vi "Controller - Fire Emergency.vi"(8 "error in (no error)":errorcluster, 10 "Emergency":bool, 11 "View Model":T1) -> (0 "error out":errorcluster, 3 "View Model":T1)   [LabVIEW 2017]
doc: "Fire User Event = Emergency"
uses:
  View Model/Controls/View Model.ctl
  View Model/Controls/Shared Model.ctl
  Error/Controls/Error Model.ctl
  Error/Controls/Error Event.ctl
  Error/Controls/Error Type.ctl
  Configuration/Controls/Config DB Model.ctl
  Configuration/Controls/Config DB Command.ctl
  Configuration/Controls/Config DB Record.ctl
  Controls/Controller Model.ctl
  Controls/Elevator Location.ctl
  Controls/Elevator Direction Event.ctl
  Controls/Elevator Direction.ctl
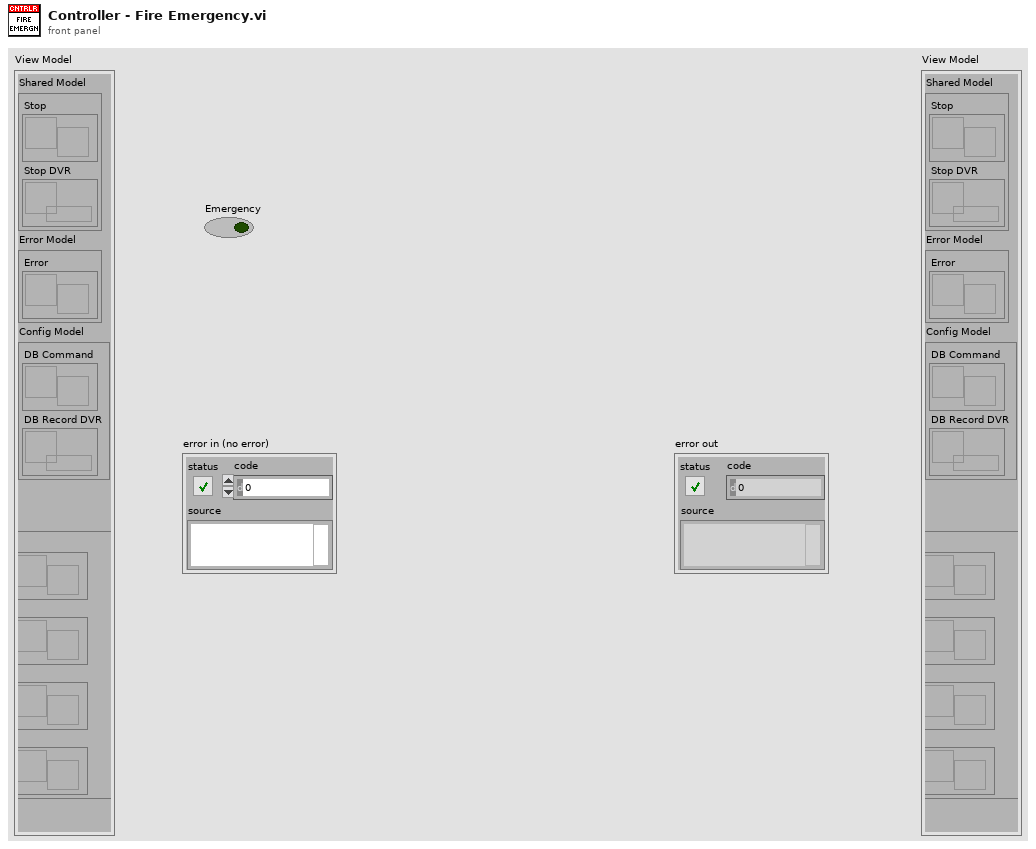
[diagram p1: front panel]
types:
  T1 = typedef "View Model.ctl" = cluster{"Shared Model":T2, "Error Model":T3, "Config Model":T4, "Controller Model":T5}
  T2 = typedef "Shared Model.ctl" = cluster{"Stop":refnum<user-event>, "Stop DVR":refnum<data-value>}
  T3 = typedef "Error Model.ctl" = cluster{"Error":refnum<user-event>}
  T4 = typedef "Config DB Model.ctl" = cluster{"DB Command":refnum<user-event>, "DB Record DVR":refnum<data-value>}
  T5 = typedef "Controller Model.ctl" = cluster{"Go to Floor":refnum<user-event>, "Emergency":refnum<user-event>, "Open/Close Door":refnum<user-event>, "Move To":refnum<user-event>}
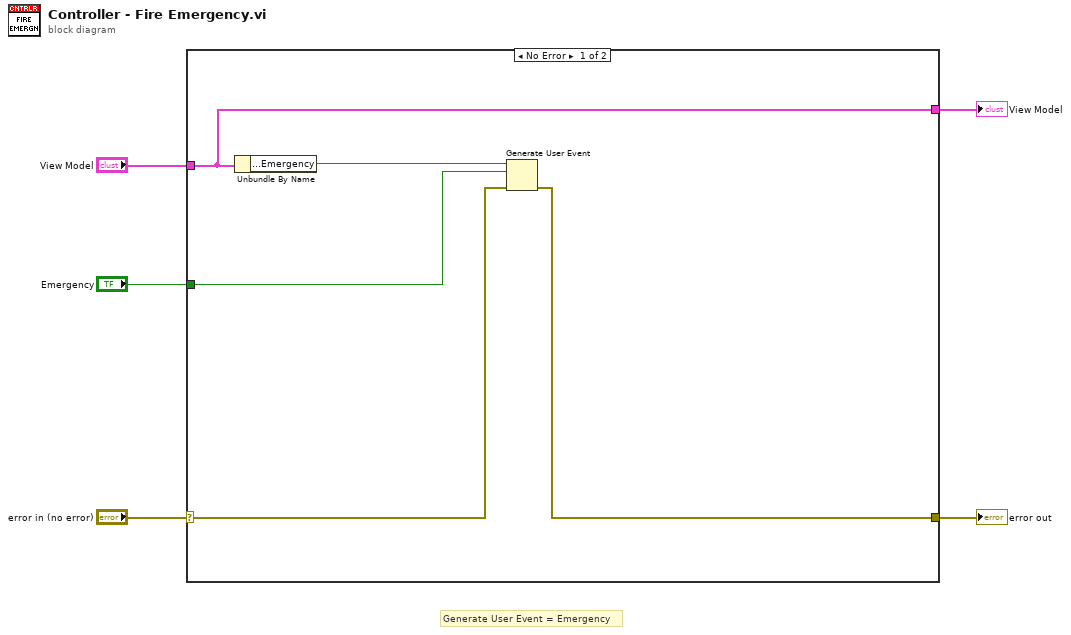
[diagram p0: block diagram]
diagram:
  # "Generate User Event = Emergency"
  n1 = case shown="No Error" "error in (no error)" {
    selector: "error in (no error)" -> [w9 w11]
    tunnel: "View Model" -> [w7 w12]
    tunnel: [w7 w12] -> w3
    tunnel: [w8 w11] -> w2
    tunnel: "Emergency" -> [w6 _]
    frame No Error {
      n2 = Unbundle By Name(w7) -> ("Controller Model.Emergency"=w10:refnum<user-event>)
      n3 = Generate User Event(user event=w10, event data cluster=w6, error in=w9) -> (error out=w8:errorcluster)  [unwired: 1 in, 1 out]
    }
    frame Error {
    }
  }
  "error out" <- w2
  "View Model" <- w3
